vi "DecodificaAO_new.vi"(4 "ForzaAO_PLC":refnum<vi>, 6 "ForzaAO_Cdaq":refnum<vi>, 7 "Caratteristiche Caricate":string[][](array[string]), 8 "AO non scalati IN":T5, 9 "AO PLCs in":T4, 10 "statoAO_Cdaq in":T9, 11 "Cluster SET AO":T6) -> (0 "AO PLCs out":T4, 1 "exit":bool, 3 "statoAO_Cdaq out":T9, 5 "AO non scalati OUT":T5)   [LabVIEW 2019]
uses:
  cDAQ/AO List.ctl
  GlobalAOInterfaccia.vi
  GlobalForzaUscite.vi
  Global config keb.vi
  Global dati targa SINUSPENTA.vi
  controls/statoAO_plc_1.ctl
  controls/StatoAO_cdaq.ctl
  cDAQ/SET SINGLE AO.ctl
  cDAQ/SET ARRAY AO.ctl
  TypeDef/Lista AO sistema.ctl
  controls/statoAO_plc_2.ctl
  controls/statoAO_plc_3.ctl
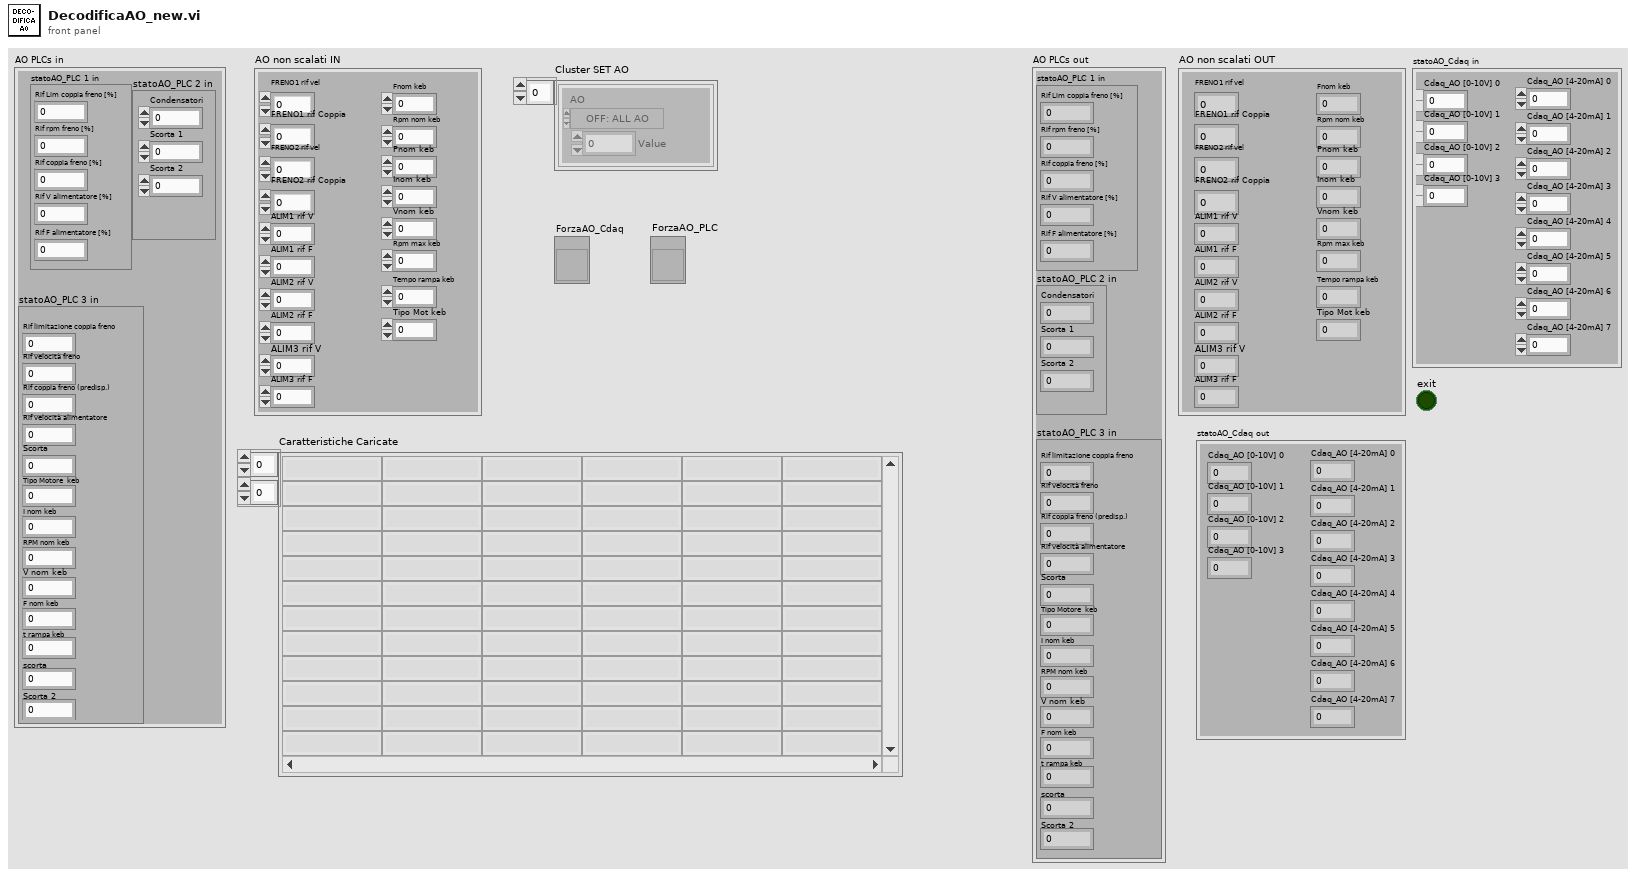
[diagram p1: front panel]
types:
  T1 = typedef "statoAO_plc_1.ctl" = cluster{"Rif Lim coppia freno [%]":dbl, "Rif rpm freno [%]":dbl, "Rif coppia freno [%]":dbl, "Rif V alimentatore [%]":dbl, "Rif F alimentatore [%]":dbl}
  T2 = typedef "statoAO_plc_2.ctl" = cluster{"Condensatori":dbl, "Scorta 1":dbl, "Scorta 2":dbl}
  T3 = typedef "statoAO_plc_3.ctl" = cluster{"Rif limitazione coppia freno":dbl, "Rif velocità freno":dbl, "Rif coppia freno (predisp.)":dbl, "Rif velocità alimentatore":dbl, "Scorta":dbl, "Tipo Motore  keb":dbl, "I nom keb":dbl, "RPM nom keb":dbl, "V nom keb":dbl, "F nom keb":dbl, "t rampa keb":dbl, "scorta":dbl, "Scorta 2":dbl}
  T4 = cluster{"statoAO_PLC 1 in":T1, "statoAO_PLC 2 in":T2, "statoAO_PLC 3 in":T3}
  T5 = typedef "Lista AO sistema.ctl" = cluster{"FRENO1 rif vel":dbl, "FRENO1 rif Coppia":dbl, "FRENO2 rif vel":dbl, "FRENO2 rif Coppia":dbl, "ALIM1 rif V":dbl, "ALIM1 rif F":dbl, "ALIM2 rif V":dbl, "ALIM2 rif F":dbl, "ALIM3 rif V":dbl, "ALIM3 rif F":dbl, "Fnom keb":dbl, "Rpm nom keb":dbl, "Pnom keb":dbl, "Inom keb":dbl, "Vnom keb":dbl, "Rpm max keb":dbl, "Tempo rampa keb":dbl, "Tipo Mot keb":dbl}
  T6 = typedef "SET ARRAY AO.ctl" = T7[]
  T7 = typedef "SET SINGLE AO.ctl" = cluster{"AO":T8, "Value":dbl}
  T8 = typedef "AO List.ctl" = enum16{"OFF: ALL AO", "RIF VEL FRENO 1", "RIF VEL FRENO 2", "RIF VEL FRENO 3", "RIF COPPIA FRENO 1", "RIF COPPIA FRENO 2", "RIF COPPIA FRENO 3", "RIF V ALIM 1", "RIF F ALIM 1", "RIF V ALIM 2", "RIF F ALIM 2", "RIF V ALIM 3", "RIF F ALIM 3", "RIF V ALIM 4", "RIF F ALIM 4", "FORZA AO PLC 3", "FORZA AO PLC 2", "FORZA AO PLC 1", "FORZA AO cDAQ", "Configura alimentatore keb", "Tempo rampa keb", "Condensatori", "Exit"}
  T9 = typedef "StatoAO_cdaq.ctl" = cluster{"Cdaq_AO [0-10V] 0":dbl, "Cdaq_AO [0-10V] 1":dbl, "Cdaq_AO [0-10V] 2":dbl, "Cdaq_AO [0-10V] 3":dbl, "Cdaq_AO [4-20mA] 0":dbl, "Cdaq_AO [4-20mA] 1":dbl, "Cdaq_AO [4-20mA] 2":dbl, "Cdaq_AO [4-20mA] 3":dbl, "Cdaq_AO [4-20mA] 4":dbl, "Cdaq_AO [4-20mA] 5":dbl, "Cdaq_AO [4-20mA] 6":dbl, "Cdaq_AO [4-20mA] 7":dbl}
  T10 = typedef "ConfigurazioneKeb.ctl" = cluster{"Freq nom":dbl, "RPM nom":dbl, "Pot nom":dbl, "I nom":dbl, "V nom":dbl, "Rpm max":dbl, "Tipo Motore":dbl}
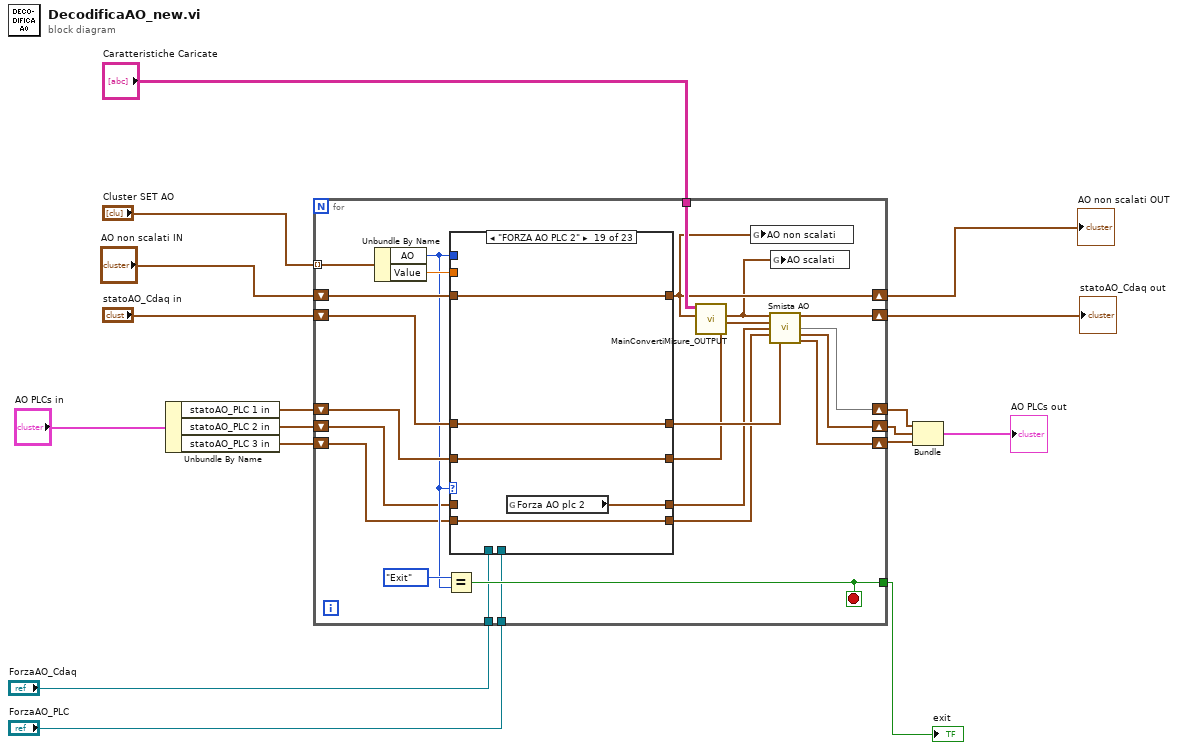
[diagram p0: block diagram]
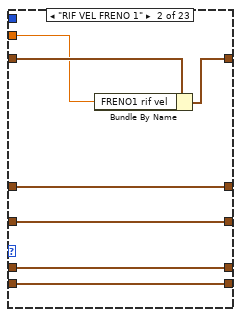
[diagram p3: hidden frame]
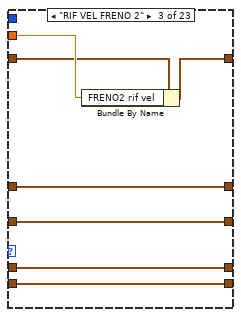
[diagram p4: hidden frame]
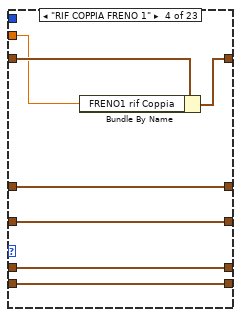
[diagram p5: hidden frame]
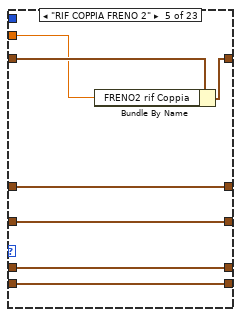
[diagram p6: hidden frame]
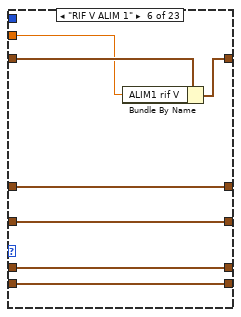
[diagram p7: hidden frame]
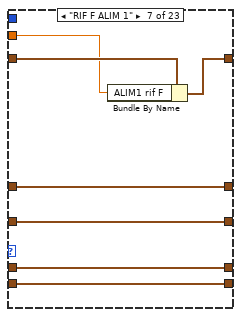
[diagram p8: hidden frame]
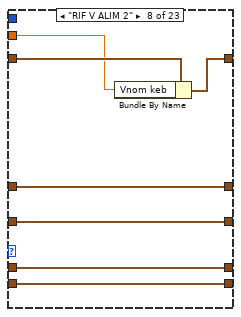
[diagram p9: hidden frame]
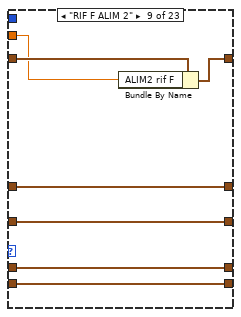
[diagram p10: hidden frame]
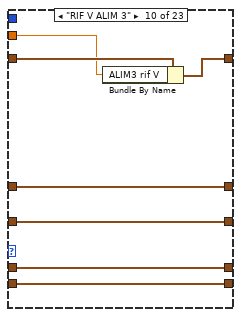
[diagram p11: hidden frame]
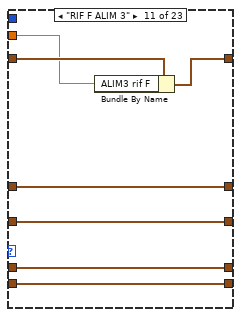
[diagram p12: hidden frame]
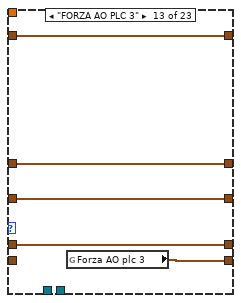
[diagram p14: hidden frame]
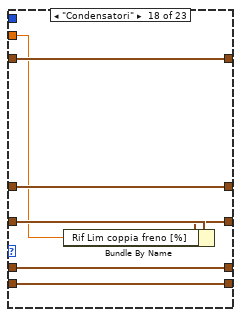
[diagram p19: hidden frame]
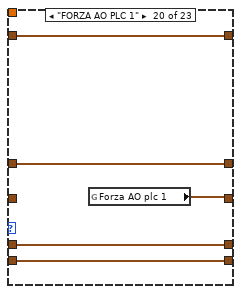
[diagram p20: hidden frame]
diagram:
  n1 = Unbundle By Name("AO PLCs in") -> ("statoAO_PLC 1 in"=w7:T1, "statoAO_PLC 2 in"=w6:T2, "statoAO_PLC 3 in"=w5:T3)
  n2 = for {
    tunnel: "Cluster SET AO" -> [w40] mode=indexing
    shift-right: [w33] -> w12
    shift-left: "statoAO_Cdaq in" -> [w32]
    shift-right: [w24] -> w4
    shift-left: w7 -> [w39]
    tunnel: [w36] -> w16
    tunnel: "ForzaAO_Cdaq" -> [w28]
    tunnel: "ForzaAO_PLC" -> [w35]
    shift-right: [w29] -> w10
    shift-left: "AO non scalati IN" -> [w34]
    tunnel: "Caratteristiche Caricate" -> [w31]
    shift-right: [w25] -> w3
    shift-left: w6 -> [w23]
    shift-right: [w26] -> w2
    shift-left: w5 -> [w21]
    stop <- w36 stop-if-true
    n3 = Unbundle By Name(w40) -> ("AO"=w30:T8, "Value"=w38:dbl)
    n4 = Equal?(x=AO_List."Exit" ("AO"), y=w30) -> (x = y?=w36:bool)
    n5 = case shown="\"FORZA AO PLC 2\"" w30 {
      tunnel: w39 -> [w44 w52 w59 w66 w73 w80 w87 w94 w101 w108 w115 w119 w122 w130 w135 w140 w145 w150 w157 _ w167 w182 w190]
      tunnel: w38 -> [_ w49 w58 w63 w71 w77 w84 w91 w98 w105 w112 _ _ _ _ _ _ w148 _ _ _ _ w184]
      tunnel: w30 -> [_ _ _ _ _ _ _ _ _ _ _ _ _ _ _ _ _ _ _ _ _ _ _]
      tunnel: w28 -> [_ _ _ _ _ _ _ _ _ _ _ _ _ _ _ _ _ _ _ _ _ _ _]
      tunnel: w35 -> [_ _ _ _ _ _ _ _ _ _ _ _ _ _ _ _ _ _ _ _ _ _ _]
      tunnel: w34 -> [w45 w51 w57 w65 w72 w79 w86 w93 w100 w107 w114 w120 w125 w128 w133 w138 w143 w151 w155 w161 w166 w178 w186]
      tunnel: [w44 w52 w59 w66 w73 w80 w87 w94 w101 w108 w115 w119 w122 w130 w135 w140 w145 w149 w157 w158 w167 w182 w190] -> w18
      tunnel: [w43 w48 w55 w62 w69 w76 w83 w90 w97 w104 w111 w118 w123 w129 w134 w139 w144 w152 w156 w162 w163 w181 w189] -> w27
      tunnel: w32 -> [w43 w48 w55 w62 w69 w76 w83 w90 w97 w104 w111 w118 w123 w129 w134 w139 w144 w152 w156 w162 _ w181 w189]
      tunnel: [w45 w50 w56 w64 w70 w78 w85 w92 w99 w106 w113 w120 w125 w128 w133 w138 w143 w151 w155 w161 w166 w177 w185] -> w29
      tunnel: w23 -> [w42 w47 w54 w61 w68 w75 w82 w89 w96 w103 w110 w117 w124 w127 w132 w137 w142 w147 _ w160 w165 w180 w188]
      tunnel: [w42 w47 w54 w61 w68 w75 w82 w89 w96 w103 w110 w117 w124 w127 w132 w137 w142 w147 w153 w160 w165 w180 w188] -> w22
      tunnel: w21 -> [w41 w46 w53 w60 w67 w74 w81 w88 w95 w102 w109 w116 _ w126 w131 w136 w141 w146 w154 w159 w164 w179 w187]
      tunnel: [w41 w46 w53 w60 w67 w74 w81 w88 w95 w102 w109 w116 w121 w126 w131 w136 w141 w146 w154 w159 w164 w179 w187] -> w20
      frame "OFF: ALL AO", Default {
      }
      frame "RIF VEL FRENO 1" {
        n6 = Bundle By Name(cluster=w51, "FRENO1 rif vel"=w49) -> (w50:T5)
      }
      frame "RIF VEL FRENO 2" {
        n7 = Bundle By Name(cluster=w57, "FRENO2 rif vel"=w58) -> (w56:T5)
      }
      frame "RIF COPPIA FRENO 1" {
        n8 = Bundle By Name(cluster=w65, "FRENO1 rif Coppia"=w63) -> (w64:T5)
      }
      frame "RIF COPPIA FRENO 2" {
        n9 = Bundle By Name(cluster=w72, "FRENO2 rif Coppia"=w71) -> (w70:T5)
      }
      frame "RIF V ALIM 1" {
        n10 = Bundle By Name(cluster=w79, "ALIM1 rif V"=w77) -> (w78:T5)
      }
      frame "RIF F ALIM 1" {
        n11 = Bundle By Name(cluster=w86, "ALIM1 rif F"=w84) -> (w85:T5)
      }
      frame "RIF V ALIM 2" {
        n12 = Bundle By Name(cluster=w93, "Vnom keb"=w91) -> (w92:T5)
      }
      frame "RIF F ALIM 2" {
        n13 = Bundle By Name(cluster=w100, "ALIM2 rif F"=w98) -> (w99:T5)
      }
      frame "RIF V ALIM 3" {
        n14 = Bundle By Name(cluster=w107, "ALIM3 rif V"=w105) -> (w106:T5)
      }
      frame "RIF F ALIM 3" {
        n15 = Bundle By Name(cluster=w114, "ALIM3 rif F"=w112) -> (w113:T5)
      }
      frame "Exit" {
      }
      frame "FORZA AO PLC 3" {
        n16 = global read "GlobalForzaUscite.vi" "Forza AO plc 3"() -> (w121:T3)
      }
      frame "RIF VEL FRENO 3" {
      }
      frame "RIF COPPIA FRENO 3" {
      }
      frame "RIF V ALIM 4" {
      }
      frame "RIF F ALIM 4" {
      }
      frame "Condensatori" {
        n17 = Bundle By Name(cluster=w150, "Rif Lim coppia freno [%]"=w148) -> (w149:T1)
      }
      frame "FORZA AO PLC 2" {
        n18 = global read "GlobalForzaUscite.vi" "Forza AO plc 2"() -> (w153:T2)
      }
      frame "FORZA AO PLC 1" {
        n19 = global read "GlobalForzaUscite.vi" "Forza AO plc 1"() -> (w158:T1)
      }
      frame "FORZA AO cDAQ" {
        n20 = global read "GlobalForzaUscite.vi" "ForzaAO_Cdaq"() -> (w163:T9)
      }
      frame "Configura alimentatore keb" {
        w168 = TRUE ("Dati targa KEB Inviati")
        n21 = global read "Global config keb.vi" "Configurazione keb"() -> (w176:T10)
        n22 = Unbundle By Name(w176) -> ("Freq nom"=w175:dbl, "RPM nom"=w174:dbl, "Pot nom"=w173:dbl, "I nom"=w172:dbl, "V nom"=w171:dbl, "Rpm max"=w170:dbl, "Tipo Motore"=w169:dbl)
        n23 = global write "Global dati targa SINUSPENTA.vi" "Tentativo invio dati KEB"(w168) -> ()
        n24 = global write "Global dati targa SINUSPENTA.vi" "Dati targa KEB Inviati"(w168) -> ()
        n25 = Bundle By Name(cluster=w178, "Fnom keb"=w175, "Rpm nom keb"=w174, "Pnom keb"=w173, "Inom keb"=w172, "Vnom keb"=w171, "Rpm max keb"=w170, "Tipo Mot keb"=w169) -> (w177:T5)
      }
      frame "Tempo rampa keb" {
        n26 = Bundle By Name(cluster=w186, "Tempo rampa keb"=w184) -> (w185:T5)
        n27 = global write "Global dati targa SINUSPENTA.vi" "Tempo rampa KEB inviato"(TRUE ("Tempo rampa SINUS inviato")) -> ()
      }
    }
    n28 = call "MainConvertiMisure_OUTPUT.vi"("AO non scalati"=w29, "Caratteristiche Caricate"=w31) -> ("AO scalati"=w19:T5)  [unwired: 9 in]
    n29 = global write "GlobalAOInterfaccia.vi" "AO non scalati"(w29) -> ()
    n30 = call "Smista AO.vi"("AO scalati IN"=w19, 5:w18, "Forza AO plc_2"=w22, "Forza AO plc_3"=w20, "Forza AO cdaq"=w27) -> ("statoAO_Cdaq out"=w33:T9, 8:w24, "statoAO_PLC 2 out"=w25:T2, "statoAO_PLC 3 out"=w26:T3)  [unwired: 7 in]
    n31 = global write "GlobalAOInterfaccia.vi" "AO scalati"(w19) -> ()
  }
  "statoAO_Cdaq out" <- w12
  "exit" <- w16
  "AO non scalati OUT" <- w10
  n32 = Bundle("statoAO_PLC 1 in"=w4, "statoAO_PLC 2 in"=w3, "statoAO_PLC 3 in"=w2) -> (→"AO PLCs out":T4)  [unwired: 1 in]
